vi "Autonomous A1 Center-EitherSwitch.vi"   [LabVIEW 2017]
uses:
  Framework/Robot Global Data.vi
types:
  T1 = typedef "Command Status Info.ctl" = cluster{"Name":string, "Status":T2, "notifier out":T3}
  T2 = typedef "Completion Status.ctl" = enum16{"Successful", "Aborted", "Incomplete"}
  T3 = typedef "Completion Notifier.ctl" = refnum<notifier>
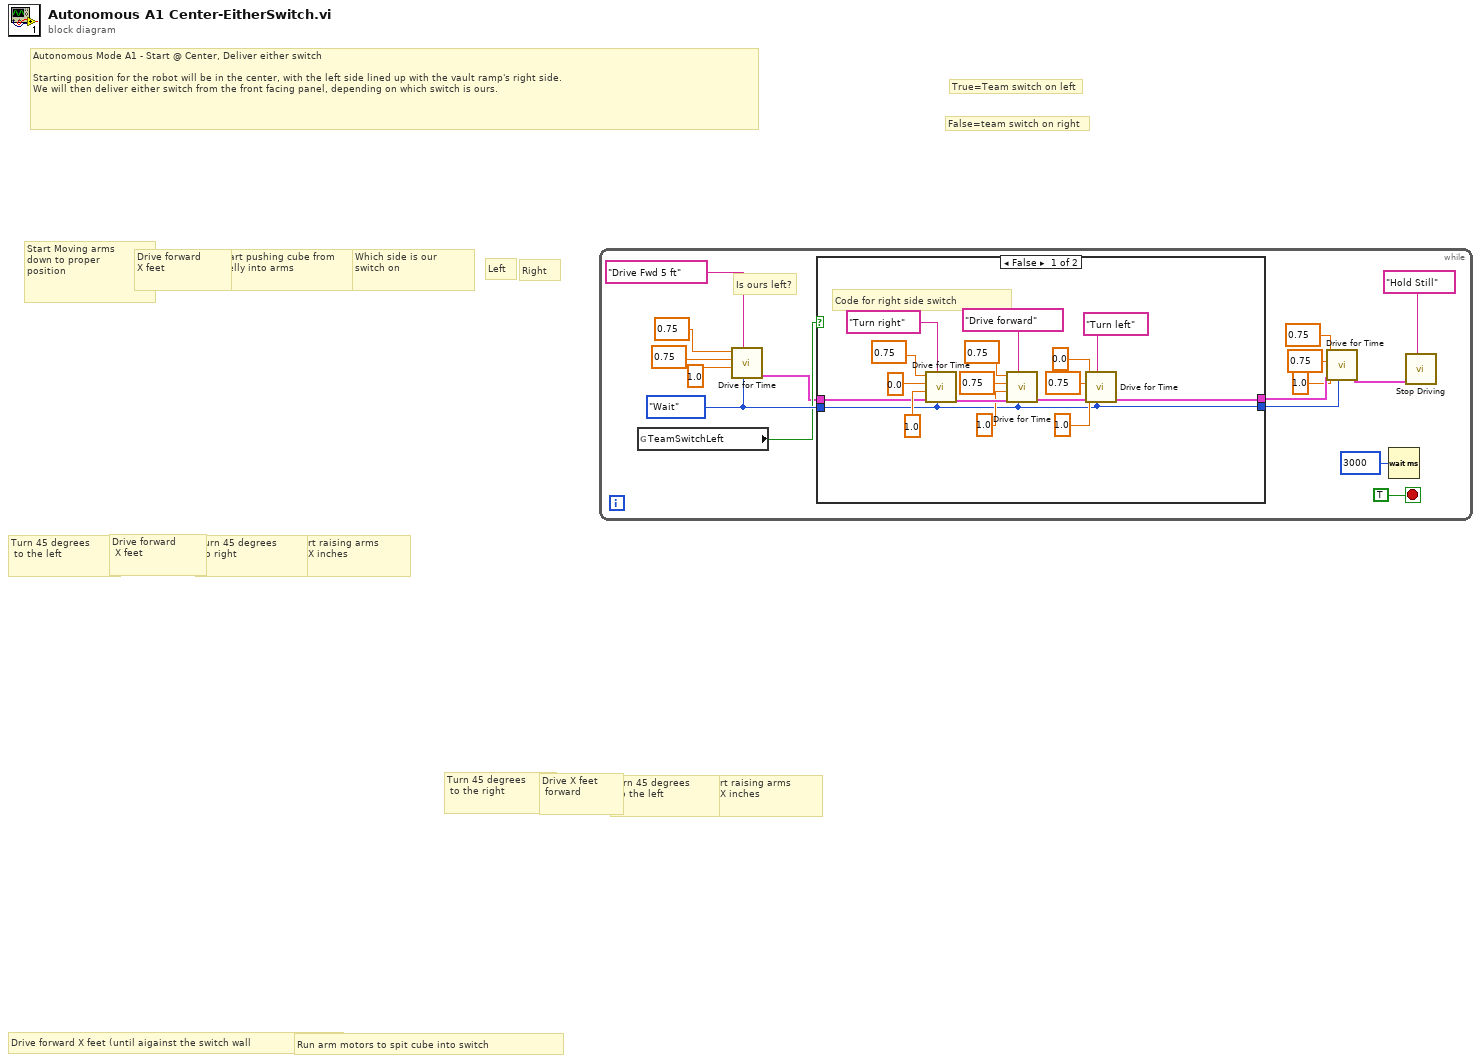
[diagram p0: block diagram]
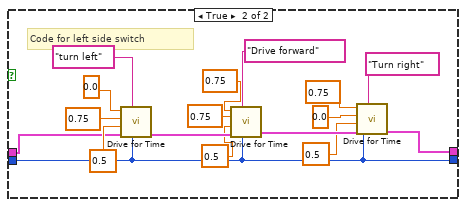
[diagram p2: hidden frame]
diagram:
  # "False=team switch on right"
  # "True=Team switch on left"
  # "Run arm motors to spit cube into switch"
  # "Drive forward X feet (until aigainst the switch wall"
  # "Start raising arms\n to X inches"
  # "turn 45 degrees\n to the left"
  # "Drive X feet\n forward"
  # "Turn 45 degrees\n to the right"
  # "Right"
  # "Start raising arms\n to X inches"
  # "Turn 45 degrees\n to right"
  # "Drive forward\n X feet"
  # "Turn 45 degrees\n to the left"
  # "Left"
  # "Which side is our \nswitch on"
  # "Start pushing cube from\n belly into arms"
  # "Drive forward\nX feet"
  # "Autonomous Mode A1 - Start @ Center, Deliver either switch\n\nStarting position for the robot will be in the center, with the left side lined up with the vault ramp's right side. \nWe will then deliver either switch from the front facing panel, depending on which switch is ours."
  # "Start Moving arms \ndown to proper \nposition"
  n1 = while {
    stop <- TRUE stop-if-true
    w4 = enum16{"Start", "Wait"}."Wait" ("Synchronication")
    # "Is ours left?"
    n2 = global read "Robot Global Data.vi" "TeamSwitchLeft"() -> (w2:bool)
    n3 = call "Drive for Time.vi"("Synchronization"=w4, "Description"="Drive Fwd 5 ft", "Seconds"=1.0 ("Delay (s)"), "Right Speed"=0.75 ("X axis value"), "Left Speed"=0.75 ("X axis value")) -> ("Command Info Out"=w1:T1)  [unwired: 5 in, 1 out]
    n4 = case shown="False" w2 {
      tunnel: w1 -> [w29 w46]
      tunnel: w4 -> [w17 w34]
      tunnel: [w18 w35] -> w9
      tunnel: [w17 w34] -> w3
      frame False {
        # "Code for right side switch"
        n5 = call "Drive for Time.vi"("Synchronization"=w17, "Description"="Turn right", "Command Info In"=w29, "Seconds"=1.0 ("Delay (s)"), "Right Speed"=0.0 ("X axis value"), "Left Speed"=0.75 ("X axis value")) -> ("Command Info Out"=w28:T1)  [unwired: 4 in, 1 out]
        n6 = call "Drive for Time.vi"("Synchronization"=w17, "Description"="Drive forward", "Command Info In"=w28, "Seconds"=1.0, "Right Speed"=0.75, "Left Speed"=0.75) -> ("Command Info Out"=w27:T1)  [unwired: 4 in, 1 out]
        n7 = call "Drive for Time.vi"("Synchronization"=w17, "Description"="Turn left", "Command Info In"=w27, "Seconds"=1.0, "Right Speed"=0.75, "Left Speed"=0.0) -> ("Command Info Out"=w18:T1)  [unwired: 4 in, 1 out]
      }
      frame True {
        # "Code for left side switch"
        n8 = call "Drive for Time.vi"("Synchronization"=w34, "Description"="turn left", "Command Info In"=w46, "Seconds"=0.5 ("Delay (s)"), "Right Speed"=0.75 ("X axis value"), "Left Speed"=0.0 ("X axis value")) -> ("Command Info Out"=w45:T1)  [unwired: 4 in, 1 out]
        n9 = call "Drive for Time.vi"("Synchronization"=w34, "Description"="Drive forward", "Command Info In"=w45, "Seconds"=0.5, "Right Speed"=0.75, "Left Speed"=0.75) -> ("Command Info Out"=w41:T1)  [unwired: 4 in, 1 out]
        n10 = call "Drive for Time.vi"("Synchronization"=w34, "Description"="Turn right", "Command Info In"=w41, "Seconds"=0.5, "Right Speed"=0.0, "Left Speed"=0.75) -> ("Command Info Out"=w35:T1)  [unwired: 4 in, 1 out]
      }
    }
    n11 = call "Drive for Time.vi"("Synchronization"=w3, "Command Info In"=w9, "Seconds"=1.0, "Right Speed"=0.75, "Left Speed"=0.75) -> ("Command Info Out"=w5:T1)  [unwired: 5 in, 1 out]
    n12 = Wait (ms)(milliseconds to wait=u32 3000 ("millisecond timer value")) -> ()  [unwired: 1 out]
    n13 = call "Stop Driving.vi"("Description"="Hold Still", "Command Info In"=w5) -> ()  [unwired: 9 in, 1 out]
  }
